vi "功能试验.vi"(8 "error in (no error)":errorcluster caption="错误输入（无错误）", 11 "信号数据":dbl[][](array[numeric])) -> (0 "error out":errorcluster caption="错误输出")   [LabVIEW 2015, in "Logging.lvlib"]
uses:
  Logging.lvlib
panel:
  out "反转扭矩变化峰值":dbl
  out "反转最小值":dbl
  out "反转最大值":dbl
  out "扭矩反转平均值":dbl
  out "左右变化值":dbl
  out "正转扭矩变化峰值":dbl
  out "正转最小值":dbl
  out "正转最大值":dbl
  out "扭矩正转平均值":dbl
  out "总圈数":dbl
  in  "取消按钮":bool
  in  "确定按钮":bool
  # "功能测量结果"
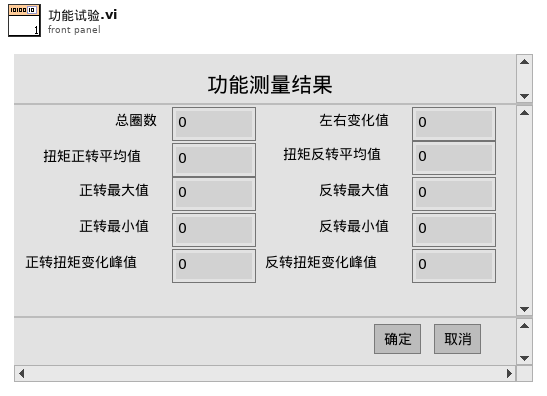
[diagram p1: front panel]
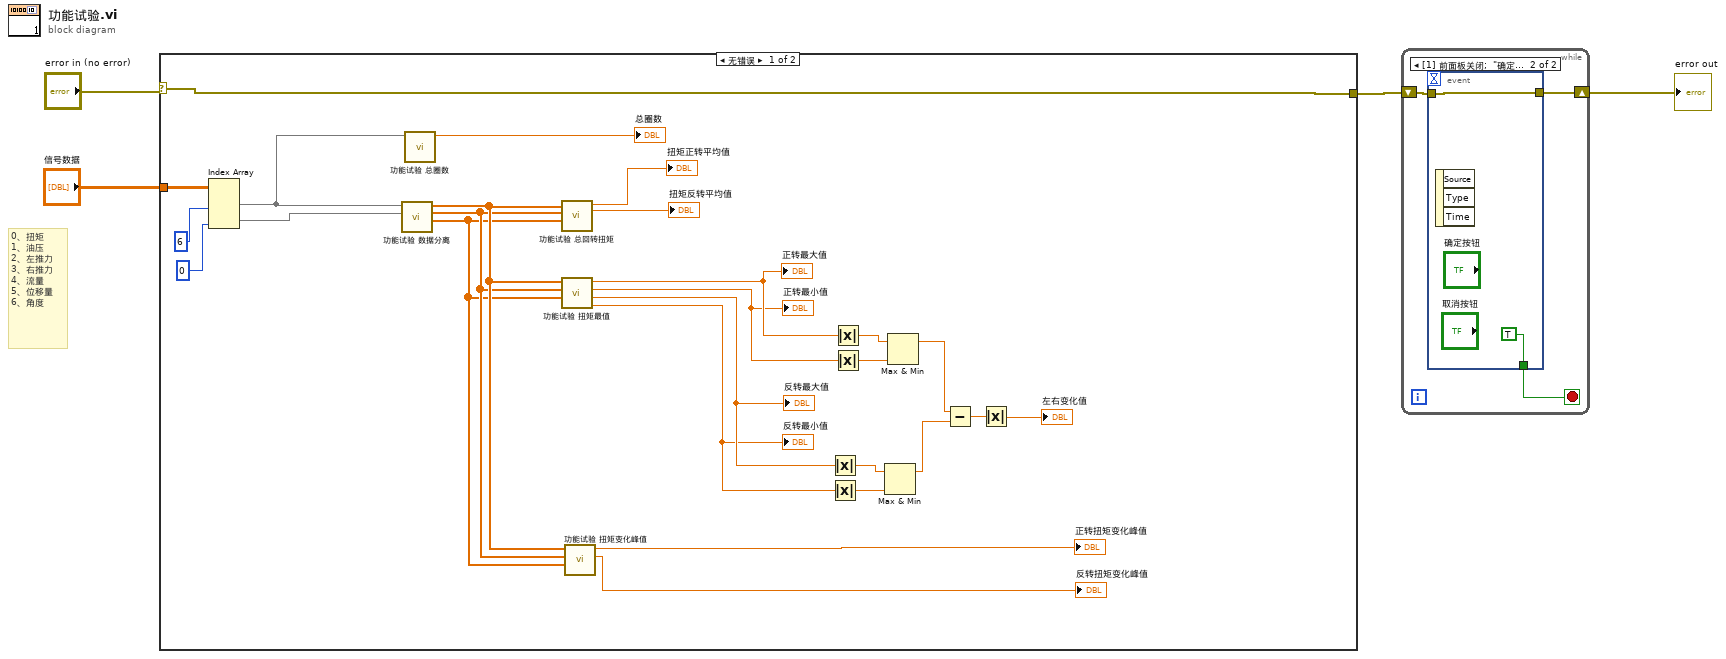
[diagram p0: block diagram]
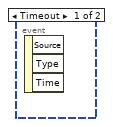
[diagram p2: hidden frame]
diagram:
  # "0、扭矩\n1、油压\n2、左推力\n3、右推力\n4、流量\n5、位移量\n6、角度"
  n1 = case shown="无错误" "error in (no error)" {
    selector: "error in (no error)" -> [w7 w31]
    tunnel: "信号数据" -> [w30 _]
    tunnel: [w7 w31] -> w1
    frame No Error {
      n2 = Index Array(array=w30, index (col) #1=6 ("禁用的索引 (列)"), index (col) #2=0 ("索引 (行)")) -> (element #1=w28:dbl[], element #2=w29:dbl[])  [unwired: 2 in]
      n3 = call "功能试验 数据分离.vi"("扭矩"=w29, "角度"=w28) -> ("扭矩右转2"=w10:dbl[], "扭矩左转"=w11:dbl[], "扭矩右转1"=w12:dbl[])  [unwired: 7 in]
      n4 = call "功能试验 总圈数.vi"("输入角度"=w28) -> ("总圈数"=→"总圈数":dbl)  [unwired: 10 in]
      n5 = call "功能试验 总回转扭矩.vi"("扭矩正转2"=w10, "扭矩反转"=w11, "扭矩正转1"=w12) -> ("扭矩反转平均值"=→"扭矩反转平均值":dbl, "扭矩正转平均值"=→"扭矩正转平均值":dbl)  [unwired: 7 in]
      n6 = call "功能试验 扭矩最值.vi"("扭矩正转2"=w10, "扭矩反转"=w11, "扭矩正转1"=w12) -> ("反转最小值"=w17:dbl, "反转最大值"=w18:dbl, "正转最小值"=w23:dbl, "正转最大值"=w24:dbl)  [unwired: 5 in]
      "正转最大值" <- w24
      "正转最小值" <- w23
      "反转最大值" <- w18
      "反转最小值" <- w17
      n7 = call "功能试验 扭矩变化峰值.vi"("扭矩正转2"=w10, "扭矩反转"=w11, "扭矩正转"=w12) -> ("反转扭矩变化峰值"=→"反转扭矩变化峰值":dbl, "正转扭矩变化峰值"=→"正转扭矩变化峰值":dbl)  [unwired: 7 in]
      n8 = Absolute Value(x=w18) -> (abs(x)=w19:dbl)
      n9 = Absolute Value(x=w17) -> (abs(x)=w20:dbl)
      n10 = Absolute Value(x=w24) -> (abs(x)=w21:dbl)
      n11 = Absolute Value(x=w23) -> (abs(x)=w22:dbl)
      n12 = Max & Min(x=w19, y=w20) -> (max(x,y)=w15:dbl)  [unwired: 1 out]
      n13 = Max & Min(x=w21, y=w22) -> (max(x,y)=w16:dbl)  [unwired: 1 out]
      n14 = Subtract(x=w16, y=w15) -> (x-y=w14:dbl)
      n15 = Absolute Value(x=w14) -> (abs(x)=→"左右变化值":dbl)
    }
    frame Error {
    }
  }
  n16 = while {
    shift-right: [w34] -> w2
    shift-left: w1 -> [w33]
    stop <- w32 stop-if-true
    n17 = event shown="[1] 前面板关闭;  \"确定按钮\", \"取消按钮\": 值改变" {
      selector: _ -> [_ _]
      dyn-events: _ -> [_ _]
      timeout: _ -> [_ _]
      tunnel: [_ w36] -> w34
      tunnel: w33 -> [_ w36]
      tunnel: [_ TRUE] -> w32
      event Timeout {
        n18 = event-data() -> ()  [unwired: 1 in, 3 out]
      }
      event Panel Close; "确定按钮", "取消按钮": Value Change {
        n19 = event-data() -> ()  [unwired: 1 in, 3 out]
      }
    }
  }
  "error out" <- w2
